vi "Configure Limit Test Null Offset.vi"(6 "Auto Null Offset (F: Disable)":bool, 7 "Enable Null Offset (F: Disable)":bool, 8 "error in (no error)":errorcluster, 9 "Limit Test Null Offset (0)":dbl, 10 "Channel (1: Channel 1)":i32(ring)=1 items=["Channel 1"=1, "Channel 2"=2], 11 "VISA resource name":refnum<visa-resource-name>) -> (0 "error out":errorcluster, 3 "VISA resource name out":refnum<visa-resource-name>)   [LabVIEW 2012, in "Keysight B2980 Series.lvlib"]
doc: "Configures the null offset value used for calculating the limit test data."
uses:
  Keysight B2980 Series.lvlib
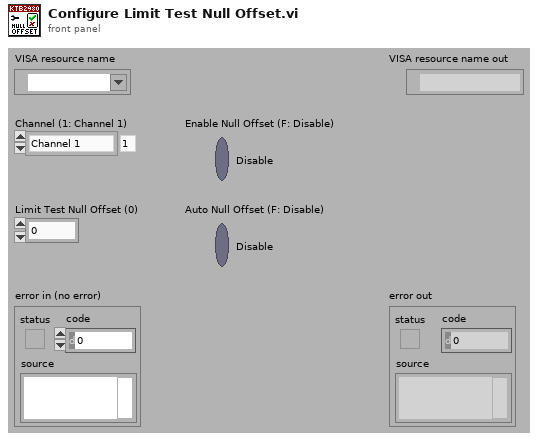
[diagram p1: front panel]
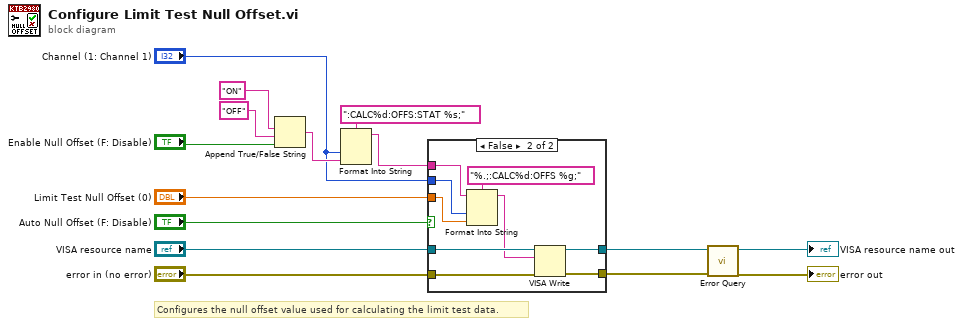
[diagram p0: block diagram]
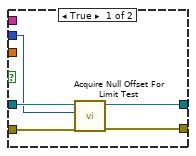
[diagram p2: hidden frame]
diagram:
  # "Configures the null offset value used for calculating the limit test data."
  n1 = Append True/False String(1:"Enable Null Offset (F: Disable)", 2:"OFF", 3:"ON") -> (0:w10:string)  [unwired: 1 out]
  n2 = Format Into String(format string=":CALC%d:OFFS:STAT %s;", "Channel (1: Channel 1)", w10) -> (resulting string=w1:string)  [unwired: 2 in, 1 out]
  n3 = case shown="False" "Auto Null Offset (F: Disable)" {
    tunnel: "Limit Test Null Offset (0)" -> [_ w28]
    tunnel: "VISA resource name" -> [w20 w27]
    tunnel: "error in (no error)" -> [w19 w25]
    tunnel: [w18 w26] -> w4
    tunnel: [w17 w24] -> w3
    tunnel: "Channel (1: Channel 1)" -> [w16 w22]
    tunnel: w1 -> [_ w21]
    frame True {
      n4 = call "Acquire Null Offset For Limit Test.vi"("error in (no error)"=w19, "Channel (1: Channel 1)"=w16, "VISA resource name"=w20) -> ("error out"=w17:errorcluster, "VISA resource name out"=w18:refnum<visa-resource-name>)  [unwired: 7 out]
    }
    frame False {
      n5 = Format Into String(format string="%.;:CALC%d:OFFS %g;", initial string=w21, w22, w28) -> (resulting string=w23:string)  [unwired: 1 in, 1 out]
      n6 = VISA Write(VISA resource name=w27, write buffer=w23, error in (no error)=w25) -> (VISA resource name out=w26:refnum<visa-resource-name>, error out=w24:errorcluster)  [unwired: 1 out]
    }
  }
  n7 = call "Error Query.vi"("error in (no error)"=w3, "VISA resource name"=w4) -> ("error out"=→"error out":errorcluster, "VISA resource name out"=→"VISA resource name out":refnum<visa-resource-name>)  [unwired: 8 out]
